vi "Initialize.vi"(2 "XRef":refnum<vi>) -> (1 "State Out":T1)   [LabVIEW 2012, in "Unindex and Unbundle.xnode"]
doc: "This ability VI is called when your XNode is first dropped. It is used to specify your initial state.\n\nDefault behavior: Intialize state to default defaults (usually zero-initialized).\n\nThis ability does not provide UI and OS messages are not handled.\n\nSee also: Copy"
uses:
  Unindex and Unbundle.xnode
  State.ctl
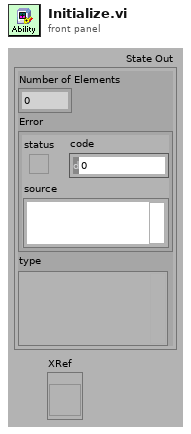
[diagram p1: front panel]
types:
  T1 = typedef "Unindex and Unbundle.xnode/State.ctl" = cluster{"Number of Elements":i32, "Error":errorcluster, "type":variant}
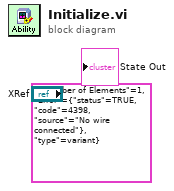
[diagram p0: block diagram]
diagram:
  "State Out" <- T1 {"Number of Elements"=1, "Error"={"status"=TRUE, "code"=4398, "source"="No wire connected"}, "type"=variant} ("State Out")
